vi "Write DataFifo.vi"(8 "error in (no error)":errorcluster, 10 "DataFifo":T1={"ReadPointer"=0, "WritePointer"=0, "Locked"=FALSE, "FifoSize"=3600}, 11 "PmuBase in":refnum<class "PmuBase.lvclass">) -> (0 "error out":errorcluster, 3 "PmuBase out":refnum<class "PmuBase.lvclass">)   [LabVIEW 2014, in "SensorPlugins.lvlib" / "PmuBase.lvclass"]
uses:
  PmuBase.lvclass
  Typedef/DataFifo.ctl
  PmuBase.lvclass/PmuBase.ctl
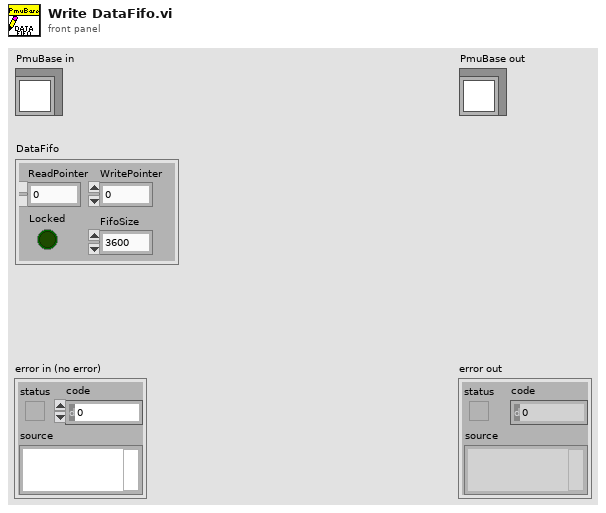
[diagram p1: front panel]
types:
  T1 = typedef "SensorPlugins.lvlib/PmuBase.lvclass/DataFifo.ctl" = cluster{"ReadPointer":u16, "WritePointer":u64, "Locked":bool, "FifoSize":u64}
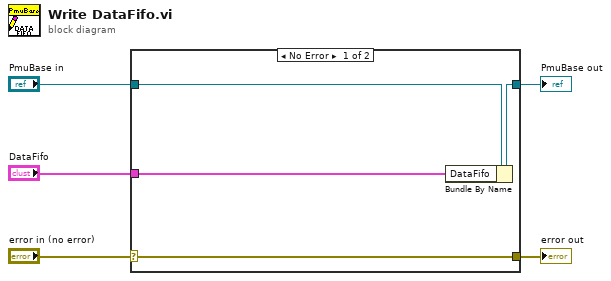
[diagram p0: block diagram]
diagram:
  n1 = case shown="No Error" "error in (no error)" {
    selector: "error in (no error)" -> [w9 w10]
    tunnel: [w9 w10] -> w4
    tunnel: [w7 w11] -> w2
    tunnel: "PmuBase in" -> [w8 w11]
    tunnel: "DataFifo" -> [w6 _]
    frame No Error {
      n2 = Bundle By Name(cluster=w8, "DataFifo"=w6) -> (w7:refnum<class "PmuBase.lvclass">)
    }
    frame Error {
    }
  }
  "error out" <- w4
  "PmuBase out" <- w2
